vi "Offline_BassShaker.vi"() -> ()   [LabVIEW 2010]
uses:
  <vilib>/Utility/error.llb/DialogType.ctl
  Types/TYPE Filter Outputs.ctl
  <vilib>/Utility/file.llb/Write To Spreadsheet File (DBL).vi
panel:
  in  "Sleep-Wake Feature:":u16(ring) items=["EMG", "Piezo", ""]
  in  "Stop":bool
  out "Loop Count":i32=84969
  in  "Data File":path=path "C:/Users/Sunderam Lab/Desktop/Sleep Modulation HMM/NSL11/NSL11_20160107_24Hr.tdms"
  out "Stim":bool
  out "Detect":bool
  in  "Target State":u16(ring)=3 items=["Wake"=1, "NREM"=2, "REM"=3]
  in  "Preamp Gain":dbl(ring)=10.0 items=["10X"=10.0, "100X"=100.0]
  in  "Min Duration":dbl=5.0
  in  "Stim":bool=TRUE
  in  "Feature Save To Path":path=path "C:/Users/Sunderam Lab/Desktop/Features.csv"
  in  "EEG Coefficients File":path=path "C:/Users/Sunderam Lab/Desktop/Sleep Modulation HMM/EEG_Coefs.csv"
  in  "Cluster Information File":path=path "C:/Users/Sunderam Lab/Desktop/Sleep Modulation HMM/Model_NSL11_20160107_24Hr.csv"
  out "Sleep Stage":i32=1
  out "EEG":waveform(dbl)(graph)={"t0"=timestamp(3543011656.0392275 s since 1904-01-01), "dt"=0.0025, "Y"=array[400 elements], "attributes"=variant("NI_ChannelName"=variant(string "EEG"), "NI_UnitDescription"=variant(string "Volts"))}
  out "EMG":waveform(dbl)(graph)={"t0"=timestamp(3543011656.0392413 s since 1904-01-01), "dt"=0.0025, "Y"=array[400 elements], "attributes"=variant("NI_ChannelName"=variant(string "EMG"), "NI_UnitDescription"=variant(string "Volts"))}
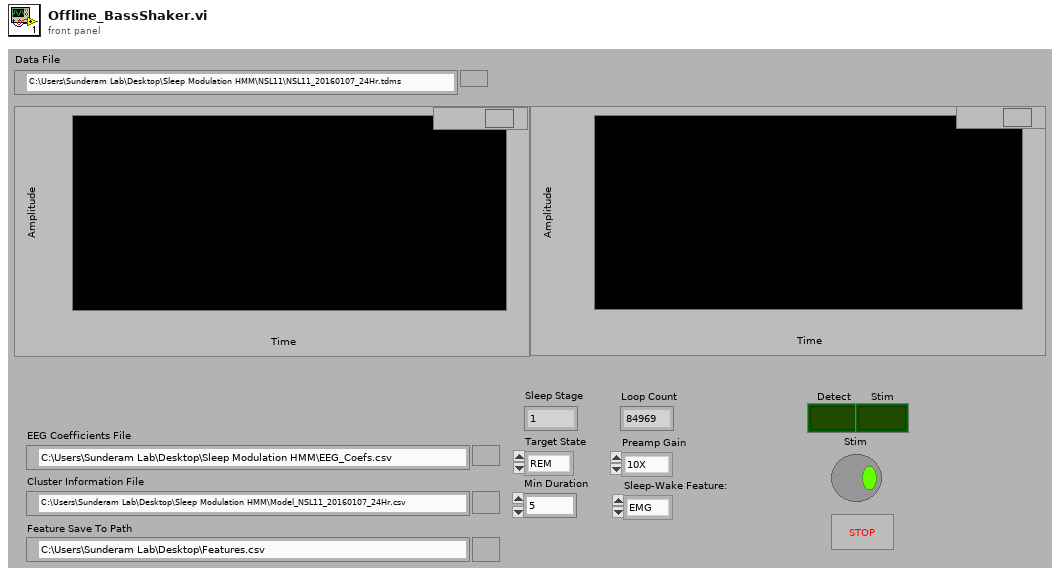
[diagram p1: front panel]
types:
  T1 = typedef "DialogType.ctl" = u16
  T2 = typedef "TYPE Filter Outputs.ctl" = cluster{"Delta:Theta":dbl, "Hi:Lo":dbl, "EMG":dbl, "Delta Low":dbl, "Theta":dbl, "Alpha":dbl, "Beta":dbl, "Gamma":dbl, "Total EEG":dbl, "Detection":dbl, "Stimulate":dbl, "TimeStamp":dbl, "Class Labels":dbl, "Delta High":dbl}
  T3 = typedef "TYPE EEG Components.ctl" = cluster{"Total":dbl, "Alpha":dbl, "Beta":dbl, "Gamma":dbl, "Delta":dbl, "Delta Low":dbl, "Delta High":dbl, "Theta":dbl}
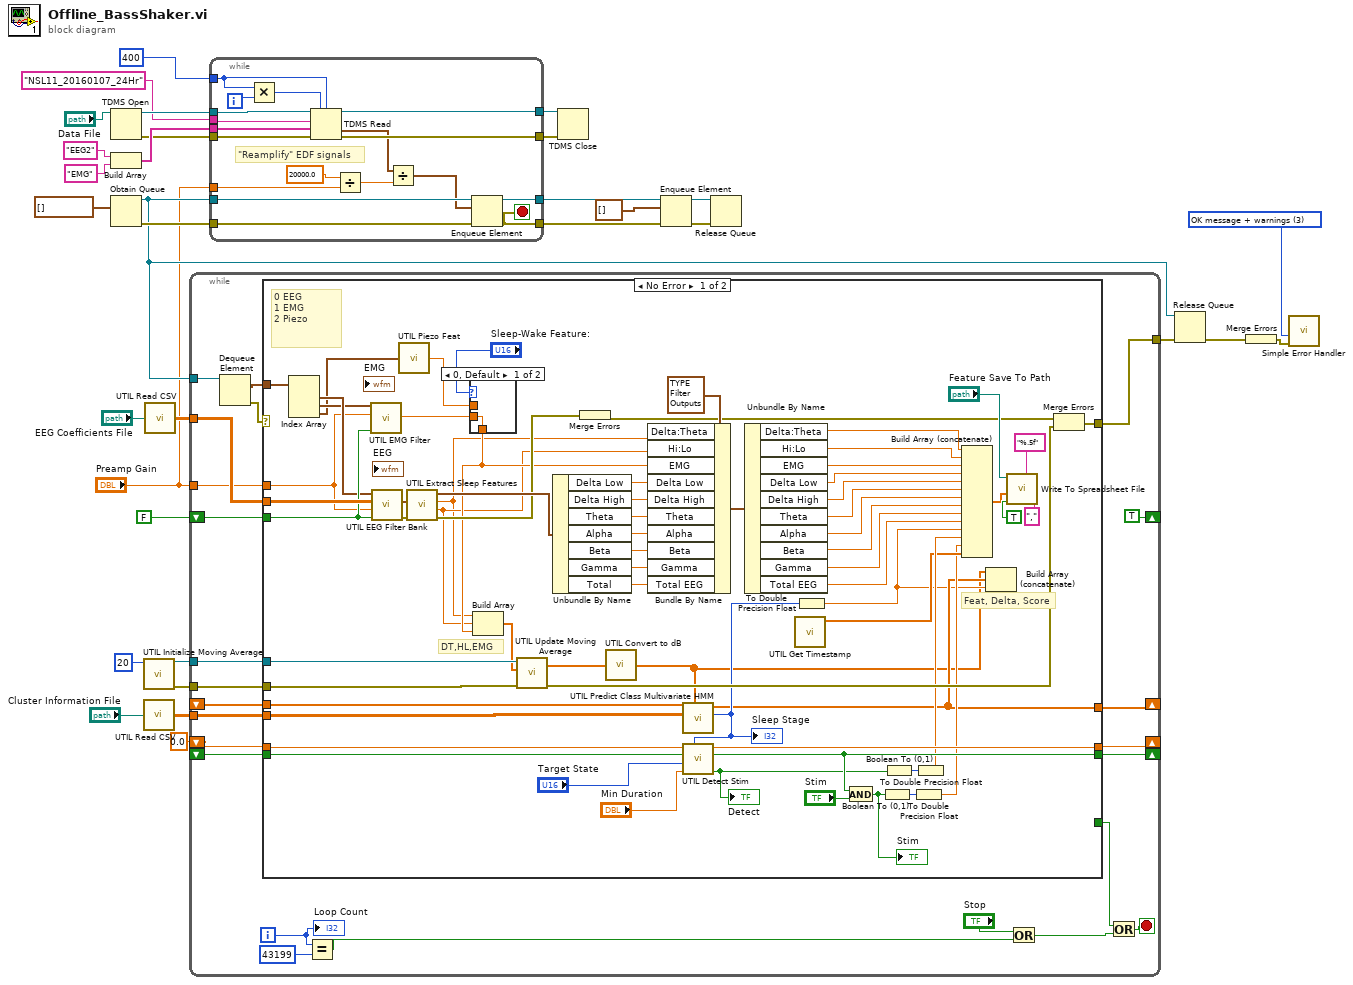
[diagram p0: block diagram]
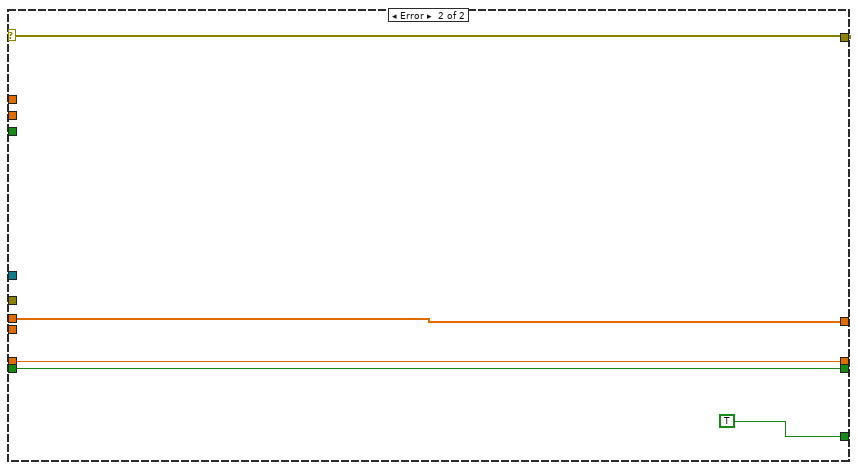
[diagram p3: hidden frame]
diagram:
  w31 = T1 3 items=["no dialog", "OK message", "continue or stop message", "OK message + warnings", "continue/stop + warnings"] ("type of dialog (OK msg:1)")
  n1 = TDMS Open(11:"Data File") -> (0:w12:errorcluster, 3:w11:refnum<k34>)  [unwired: 5 in]
  n2 = Build Array("EEG2" ("channel name"), "EMG" ("channel name")) -> (w13:string[])
  n3 = Obtain Queue(element data type=waveform(dbl)[] [] ("Measurement 2")) -> (queue out=w2:refnum<queue>, error out=w8:errorcluster)  [unwired: 4 in, 1 out]
  n4 = call "UTIL Initialize Moving Average.vi"("Window Width"=20) -> ("Error Out"=w25:errorcluster, "queue out"=w23:refnum<queue>)  [unwired: 9 in]
  n5 = call "UTIL Read CSV.vi"("CSV Path"="Cluster Information File") -> ("Data From File"=w28:dbl[][])
  n6 = call "UTIL Read CSV.vi"("CSV Path"="EEG Coefficients File") -> ("Data From File"=w22:dbl[][])
  n7 = while {
    tunnel: w2 -> [w54]
    shift-right: [TRUE] -> _
    shift-left: FALSE -> [w52]
    tunnel: [w46] -> w30
    tunnel: w25 -> [w49]
    tunnel: w28 -> [w48]
    tunnel: w22 -> [w47]
    tunnel: w23 -> [w45]
    shift-right: [w44] -> _
    shift-left: _ -> [w43]
    shift-right: [w41] -> _
    shift-left: 0.0 ("element") -> [w42]
    shift-right: [w40] -> _
    shift-left: _ -> [w39]
    tunnel: "Preamp Gain" -> [w33]
    i -> [w37]
    stop <- w51 stop-if-true
    n8 = Dequeue Element(queue=w54) -> (element=w55:waveform(dbl)[], error out=w56:errorcluster)  [unwired: 2 in, 2 out]
    n9 = case shown="No Error" w56 {
      selector: w56 -> [_ w130]
      tunnel: w55 -> [w121 _]
      tunnel: w52 -> [w96 _]
      tunnel: [_ TRUE] -> w50
      tunnel: [w99 w130] -> w46
      tunnel: w49 -> [w93 _]
      tunnel: w48 -> [w109 _]
      tunnel: w47 -> [w98 _]
      tunnel: w45 -> [w91 _]
      tunnel: [w66 w129] -> w44
      tunnel: w43 -> [w90 w129]
      tunnel: w42 -> [w83 w128]
      tunnel: [w85 w128] -> w41
      tunnel: [w80 w127] -> w40
      tunnel: w39 -> [w84 w127]
      tunnel: w33 -> [w67 _]
      frame No Error {
        # "Feat, Delta, Score"
        # "0 EEG\n1 EMG\n2 Piezo"
        # "DT,HL,EMG"
        n10 = Index Array(array=w121) -> (element #1=w95:waveform(dbl), element #2=w94:waveform(dbl), element #3=w79:waveform(dbl))  [unwired: 3 in]
        n11 = call "UTIL EMG Filter.vi"("init/cont (init:F)"=w96, "Preamp Gain"=w67, "EMG In"=w94) -> ("EMG Power"=w89:dbl)  [unwired: 7 in, 1 out]
        n12 = call "UTIL EEG Filter Bank.vi"("init/cont (init:F)"=w96, "Amplifier Gain"=w67, "Filter Coefficients from File"=w98, "EEG In"=w95) -> ("Error Out"=w124:errorcluster, "EEG Components"=w97:T3)  [unwired: 5 in, 1 out]
        n13 = call "UTIL Piezo Feat.vi"("Piezo In"=w79) -> ("Piezo Power"=w88:dbl)  [unwired: 4 in]
        n14 = call "UTIL Extract Sleep Features.vi"("Error In"=w124, "Components In"=w97) -> ("Error Out"=w110:errorcluster, "Hi:Lo"=w69:dbl, "Delta:Theta"=w68:dbl, "Components Out"=w122:T3)  [unwired: 6 in]
        n15 = case shown="0, Default" "Sleep-Wake Feature:" {
          tunnel: w89 -> [w125 _]
          tunnel: w88 -> [_ w126]
          tunnel: [w125 w126] -> w70
          frame 0, Default {
          }
          frame 1 {
          }
        }
        n16 = Build Array(w68, w69, w70) -> (w65:dbl[])
        n17 = call "UTIL Update Moving Average.vi"("Error In"=w93, "Data In"=w65, "Average Queue"=w91) -> ("Error Out"=w92:errorcluster, "Average"=w63:dbl[])  [unwired: 7 in]
        n18 = Unbundle By Name(w122) -> ("Delta Low"=w108:dbl, "Delta High"=w107:dbl, "Theta"=w106:dbl, "Alpha"=w105:dbl, "Beta"=w104:dbl, "Gamma"=w103:dbl, "Total"=w102:dbl)
        n19 = Merge Errors(w110) -> (w100:errorcluster)
        n20 = call "UTIL Convert to dB.vi"("Features In"=w63) -> ("Features (dB)"=w62:dbl[])
        n21 = Bundle By Name(cluster=T2 {"Delta:Theta"=0.0, "Hi:Lo"=0.0, "EMG"=0.0, "Delta Low"=0.0, "Theta"=0.0, "Alpha"=0.0, "Beta"=0.0, "Gamma"=0.0, "Total EEG"=0.0, "Detection"=0.0, "Stimulate"=0.0, "TimeStamp"=0.0, "Class Labels"=0.0, "Delta High"=0.0} ("Filter Outputs"), "Delta:Theta"=w68, "Hi:Lo"=w69, "EMG"=w70, "Delta Low"=w108, "Delta High"=w107, "Theta"=w106, "Alpha"=w105, "Beta"=w104, "Gamma"=w103, "Total EEG"=w102) -> (w120:T2)
        n22 = call "UTIL Predict Class Multivariate HMM.vi"("Data Point"=w62, "Model Information"=w109, "d(t-1) In"=w90) -> ("Sleep Stage"=w81:i32, "d(t-1) Out"=w66:dbl[])  [unwired: 5 in]
        "Sleep Stage" <- w81
        n23 = call "UTIL Detect Stim.vi"("Predicted State"=w81, "Min Duration"="Min Duration", "Target State"="Target State", "Previous Stim State"=w84, "Detection Duration In"=w83) -> ("Detection"=w72:bool, "Stim State Out"=w80:bool, "Detection Duration Out"=w85:dbl)  [unwired: 4 in]
        "Detect" <- w72
        n24 = Unbundle By Name(w120) -> ("Delta:Theta"=w57:dbl, "Hi:Lo"=w58:dbl, "EMG"=w59:dbl, "Delta Low"=w119:dbl, "Delta High"=w111:dbl, "Theta"=w112:dbl, "Alpha"=w113:dbl, "Beta"=w114:dbl, "Gamma"=w118:dbl, "Total EEG"=w101:dbl)
        n25 = call "UTIL Get Timestamp.vi"() -> ("appended array"=w76:dbl[])  [unwired: 7 in, 1 out]
        n26 = To Double Precision Float(number=w81) -> (double precision float=w64:dbl)
        n27 = And(x=w80, y="Stim") -> (x .and. y?=w71:bool)
        "Stim" <- w71
        n28 = Boolean To (0,1)(Boolean=w71) -> (0, 1=w75:i16)
        n29 = Boolean To (0,1)(Boolean=w72) -> (0, 1=w77:i16)
        n30 = To Double Precision Float(number=w75) -> (double precision float=w74:dbl)
        n31 = To Double Precision Float(number=w77) -> (double precision float=w78:dbl)
        n32 = Build Array (concatenate)(w57, w58, w59, w119, w111, w112, w113, w114, w118, w101, w64, w78, w74, w76) -> (w60:dbl[])
        n33 = Build Array (concatenate)(w62, w66, w64) -> ()  [unwired: 1 out]
        n34 = call-poly <vilib>:"Write To Spreadsheet File.vi"("delimiter (\\t)"="," ("delimiter (\\t)"), "format (%.3f)"="%.5f", "append to file? (new file:F)"=TRUE, "1D data"=w60, "file path (dialog if empty)"="Feature Save To Path") -> ()  [unwired: 3 in, 1 out]
        n35 = Merge Errors(w100, w92) -> (w99:errorcluster)
      }
      frame Error {
      }
    }
    n36 = Equal?(x=w37, y=43199) -> (x = y?=w36:bool)
    n37 = Or(x="Stop", y=w36) -> (x .or. y?=w34:bool)
    n38 = Or(x=w50, y=w34) -> (x .or. y?=w51:bool)
    "Loop Count" <- w37
  }
  n39 = while {
    tunnel: w11 -> [w145]
    tunnel: w12 -> [w147]
    tunnel: 400 -> [w149]
    tunnel: [w148] -> w19
    tunnel: [w146] -> w17
    tunnel: w13 -> [w144]
    tunnel: "NSL11_20160107_24Hr" ("group name") -> [w143]
    tunnel: w2 -> [w141]
    tunnel: w8 -> [w140]
    tunnel: [w139] -> w7
    tunnel: [w138] -> w6
    tunnel: "Preamp Gain" -> [w135]
    i -> [w142]
    stop <- w138 stop-if-true
    # "\"Reamplify\" EDF signals"
    n40 = Multiply(x=w149, y=w142) -> (x*y=w137:i32)
    n41 = TDMS Read(0:w145, 1:w137, 2:w149, 5:w143, 7:w144, 11:w147) -> (4:w146:refnum<k34>, 10:w133:waveform(dbl)[], 15:w148:errorcluster)  [unwired: 1 in, 3 out]
    n42 = Divide(x=20000.0, y=w135) -> (x/y=w134:dbl)
    n43 = Divide(x=w133, y=w134) -> (x/y=w132:waveform(dbl)[])
    n44 = Enqueue Element(queue=w141, element=w132, error in (no error)=w140) -> (queue out=w139:refnum<queue>, error out=w138:errorcluster)  [unwired: 1 in, 1 out]
  }
  n45 = TDMS Close(8:w19, 11:w17) -> ()  [unwired: 2 out]
  n46 = Enqueue Element(queue=w7, element=waveform(dbl)[] [] ("Measurement 2"), error in (no error)=w6) -> (queue out=w4:refnum<queue>, error out=w3:errorcluster)  [unwired: 1 in, 1 out]
  n47 = Release Queue(queue=w4, error in (no error)=w3) -> ()  [unwired: 1 in, 3 out]
  n48 = Release Queue(queue=w2, error in (no error)=w30) -> (error out=w26:errorcluster)  [unwired: 1 in, 2 out]
  n49 = Merge Errors(w26) -> (w27:errorcluster)
  n50 = call <vilib>:"Simple Error Handler.vi"("type of dialog (OK msg:1)"=w31, "error in (no error)"=w27) -> ()  [unwired: 3 in, 5 out]
